vi "Sensors Page Facade.vi"(0 "Data In":T4, 2 "Display State In":T2, 3 "Container State":T3) -> (6 "Data Out":T4, 7 "Display State Out":T2, 8 "Action":T1)   [LabVIEW 2013, in "Sensors Page X.xctl"]
uses:
  Sensors Page X.xctl
  Sensors Page Data.ctl
  Sensor DAO Class.lvclass
  <vilib>/_xctls/Container State.ctl
  Sensors Page State.ctl
  <vilib>/_xctls/Action.ctl
  Sensor DAO Class.lvclass/Sensor DAO Class.ctl
  <vilib>/Utility/miscctls.llb/LVRowAndColumnTypeDef.ctl
  <vilib>/_xctls/XControlSupport.lvlib
panel:
  in  "Sensors Table":string[][](table) caption="Sensors"
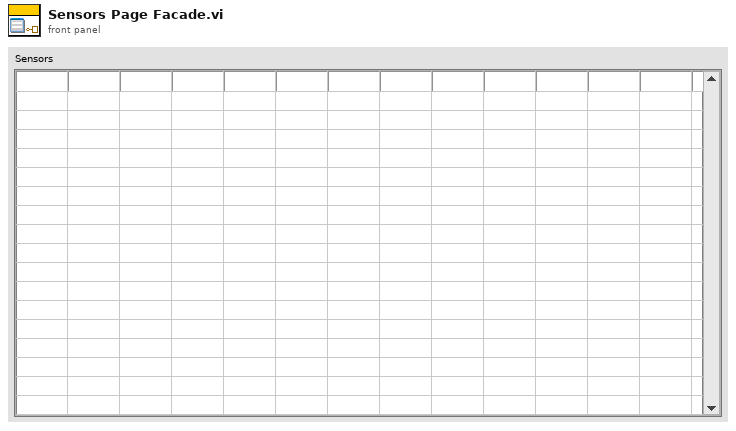
[diagram p1: front panel]
types:
  T1 = typedef "XControlSupport.lvlib/Action.ctl" = cluster{"Data Changed?":bool, "State Changed?":bool, "Action Name":string}
  T2 = typedef "Sensors Page X.xctl/Sensors Page State.ctl" = cluster{"Numeric":dbl}
  T3 = typedef "XControlSupport.lvlib/Container State.ctl" = cluster{"Indicator?":bool, "Run Mode?":bool, " Refnum":refnum<vi>}
  T4 = typedef "Sensors Page X.xctl/Sensors Page Data.ctl" = refnum<class "Sensor DAO Class.lvclass">[]
  T5 = typedef "LVRowAndColumnTypeDef.ctl" = cluster{"Row":i32, "Column":i32}
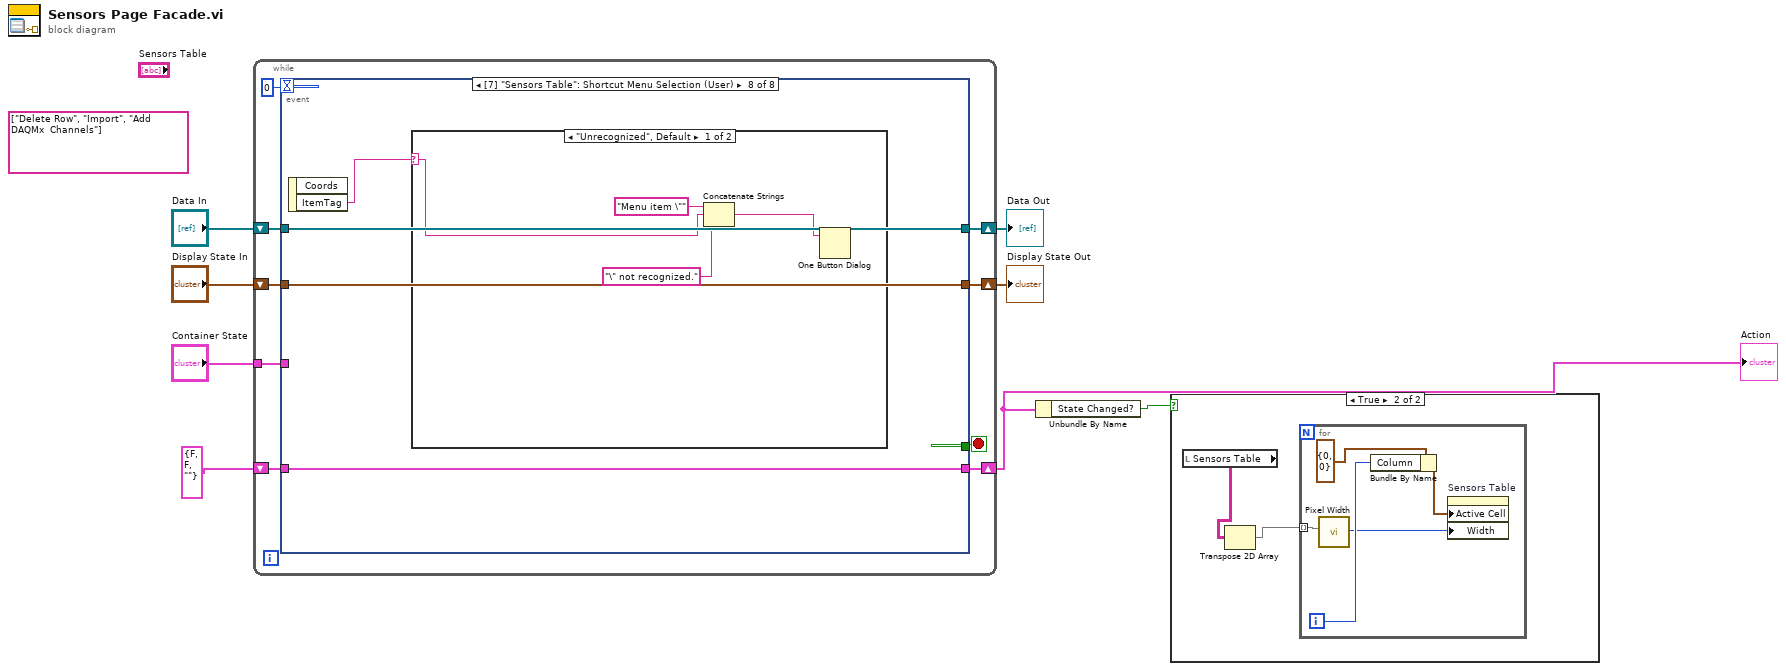
[diagram p0: block diagram]
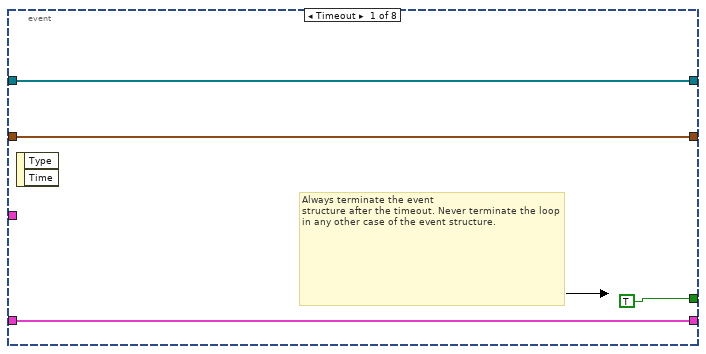
[diagram p3: hidden frame]
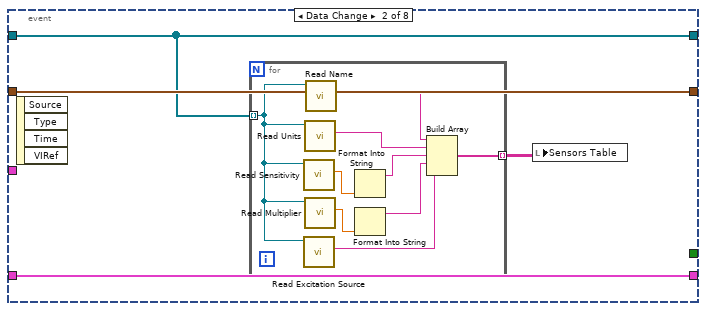
[diagram p4: hidden frame]
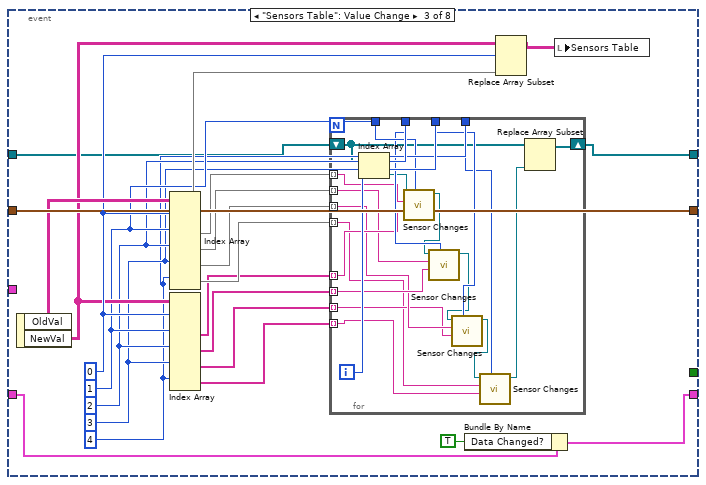
[diagram p5: hidden frame]
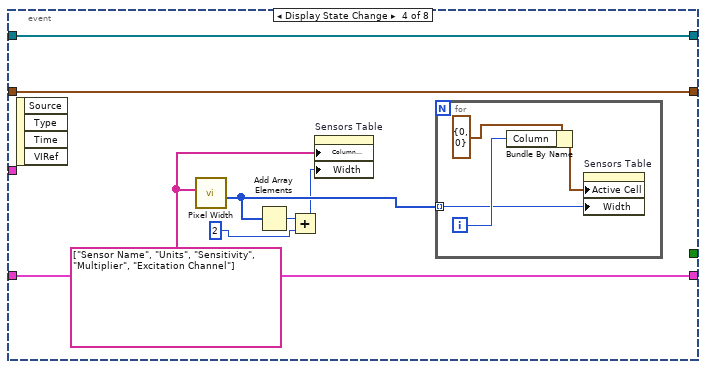
[diagram p6: hidden frame]
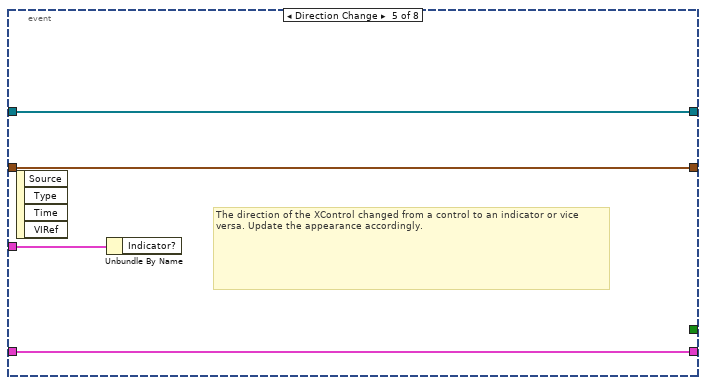
[diagram p7: hidden frame]
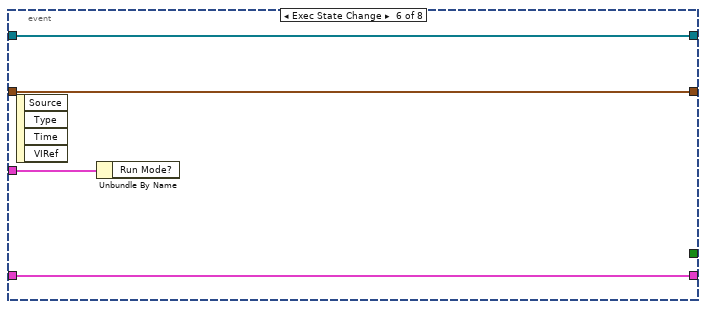
[diagram p8: hidden frame]
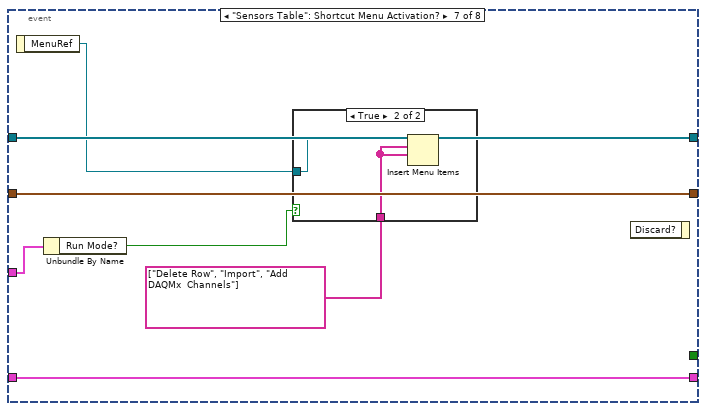
[diagram p9: hidden frame]
diagram:
  (unwired) string[] ["Delete Row", "Import", "Add DAQMx  Channels"]
  n1 = while {
    shift-right: [w16] -> w5
    shift-left: "Display State In" -> [w17]
    tunnel: "Container State" -> [w13]
    shift-right: [w11] -> w8
    shift-left: "Data In" -> [w12]
    shift-right: [w9] -> w2
    shift-left: T1 {"Data Changed?"=FALSE, "State Changed?"=FALSE, "Action Name"=""} ("Action") -> [w10]
    stop <- w15 stop-if-true
    n2 = event shown="[7] \"Sensors Table\": Shortcut Menu Selection (User)" {
      selector: _ -> [_ _ _ _ _ _ _ _]
      dyn-events: _ -> [_ _ _ _ _ _ _ _]
      timeout: 0 -> [_ _ _ _ _ _ _ _]
      tunnel: w17 -> [w19 w25 w57 w85 w92 w96 w104 w110]
      tunnel: [w19 w25 w57 w85 w92 w96 w104 w110] -> w16
      tunnel: [TRUE _ _ _ _ _ _ _] -> w15
      tunnel: w13 -> [_ _ _ _ w93 w97 w100 _]
      tunnel: w12 -> [w18 w23 w38 w84 w91 w95 w103 w109]
      tunnel: [w18 w23 w35 w84 w91 w95 w103 w109] -> w11
      tunnel: [w20 w24 w37 w83 w90 w94 w102 w108] -> w9
      tunnel: w10 -> [w20 w24 w56 w83 w90 w94 w102 w108]
      event Timeout {
        # "Always terminate the event\nstructure after the timeout. Never terminate the loop in any other case of the event structure."
        n3 = event-data() -> ()  [unwired: 1 in, 2 out]
      }
      event Data Change {
        n4 = event-data() -> ()  [unwired: 1 in, 4 out]
        n5 = for {
          tunnel: w23 -> [w34] mode=indexing
          tunnel: [w26] -> w22 mode=indexing
          n6 = call "Read Sensitivity.vi"("Sensor DAO Class in"=w34) -> ("Sensitivity"=w33:dbl)  [unwired: 8 in, 2 out]
          n7 = call "Read Excitation Source.vi"("Sensor DAO Class in"=w34) -> ("Excitation Source"=w27:string)  [unwired: 8 in, 2 out]
          n8 = call "Read Units.vi"("Sensor DAO Class in"=w34) -> ("Units"=w30:string)  [unwired: 8 in, 2 out]
          n9 = call "Read Multiplier.vi"("Sensor DAO Class in"=w34) -> ("Multiplier"=w32:dbl)  [unwired: 8 in, 2 out]
          n10 = call "Read Name.vi"("Sensor DAO Class in"=w34) -> ("Name"=w31:string)  [unwired: 8 in, 2 out]
          n11 = Format Into String(w33) -> (resulting string=w29:string)  [unwired: 3 in, 1 out]
          n12 = Format Into String(w32) -> (resulting string=w28:string)  [unwired: 3 in, 1 out]
          n13 = Build Array(w31, w30, w29, w28, w27) -> (w26:string[])
        }
        n14 = local write "Sensors Table"(w22) -> ()
      }
      event "Sensors Table": Value Change {
        w39 = 4 ("index (row)")
        w40 = 3 ("index (row)")
        w41 = 2 ("index (row)")
        w42 = 1 ("index (row)")
        w54 = 0 ("index (row)")
        n15 = event-data() -> ("OldVal"=w55:string[][], "NewVal"=w53:string[][])  [unwired: 1 in]
        n16 = Index Array(array=w55, index (row) #1=w54, index (row) #2=w42, index (row) #3=w41, index (row) #4=w40, index (row) #5=w39) -> (element #1=w52:string[], element #2=w50:string[], element #3=w49:string[], element #4=w48:string[], element #5=w47:string[])  [unwired: 5 in]
        n17 = Index Array(array=w53, index (row) #1=w54, index (row) #2=w42, index (row) #3=w41, index (row) #4=w40, index (row) #5=w39) -> (element #2=w46:string[], element #3=w45:string[], element #4=w44:string[], element #5=w43:string[])  [unwired: 5 in, 1 out]
        n18 = for {
          tunnel: w50 -> [w65] mode=indexing
          tunnel: w49 -> [w63] mode=indexing
          tunnel: w48 -> [w61] mode=indexing
          tunnel: w47 -> [w59] mode=indexing
          tunnel: w46 -> [w64] mode=indexing
          tunnel: w45 -> [w62] mode=indexing
          tunnel: w44 -> [w60] mode=indexing
          tunnel: w43 -> [w58] mode=indexing
          tunnel: w42 -> [w77]
          tunnel: w41 -> [w76]
          tunnel: w40 -> [w75]
          tunnel: w39 -> [w74]
          shift-right: [w71] -> w35
          shift-left: w38 -> [w72]
          i -> [w73]
          n19 = Index Array(array=w72, index=w73) -> (element=w70:refnum<class "Sensor DAO Class.lvclass">)
          n20 = call "Sensor Changes.vi"("Index"=w77, "New"=w64, "Old"=w65, "Sensor DAO Class In"=w70) -> ("Sensor DAO Class Out"=w69:refnum<class "Sensor DAO Class.lvclass">)  [unwired: 7 in]
          n21 = call "Sensor Changes.vi"("Index"=w76, "New"=w62, "Old"=w63, "Sensor DAO Class In"=w69) -> ("Sensor DAO Class Out"=w68:refnum<class "Sensor DAO Class.lvclass">)  [unwired: 7 in]
          n22 = call "Sensor Changes.vi"("Index"=w75, "New"=w60, "Old"=w61, "Sensor DAO Class In"=w68) -> ("Sensor DAO Class Out"=w67:refnum<class "Sensor DAO Class.lvclass">)  [unwired: 7 in]
          n23 = call "Sensor Changes.vi"("Index"=w74, "New"=w58, "Old"=w59, "Sensor DAO Class In"=w67) -> ("Sensor DAO Class Out"=w66:refnum<class "Sensor DAO Class.lvclass">)  [unwired: 7 in]
          n24 = Replace Array Subset(array=w72, new element=w66) -> (w71:T4)  [unwired: 1 in]
        }
        n25 = Bundle By Name(cluster=w56, "Data Changed?"=TRUE) -> (w37:T1)
        n26 = Replace Array Subset(array=w53, new element=w52, index (row)=w54) -> (w51:string[][])  [unwired: 1 in]
        n27 = local write "Sensors Table"(w51) -> ()
      }
      event Display State Change {
        w82 = string[] ["Sensor Name", "Units", "Sensitivity", "Multiplier", "Excitation Channel"]
        n28 = event-data() -> ()  [unwired: 1 in, 4 out]
        n29 = call "Pixel Width.vi"("Array"=w82) -> ("Widths"=w81:i32[])  [unwired: 9 in, 1 out]
        n30 = Add Array Elements(numeric array=w81) -> (sum=w80:i32)
        n31 = Add(x=w80, y=2) -> (x+y=w78:i32)
        n32 = property on="Sensors Table" class="Tbl (strict)"("Column Headers[]"=w82, "Width"=w78) -> ()  [unwired: 2 in, 2 out]
        n33 = for {
          tunnel: w81 -> [w86] mode=indexing
          i -> [w87]
          n34 = Bundle By Name(cluster=T5 {"Row"=0, "Column"=0} ("Active Cell:Active Cell"), "Column"=w87) -> (w88:T5)
          n35 = property on="Sensors Table" class="Tbl (strict)"("Active Cell"=w88, "Width"=w86) -> ()  [unwired: 2 in, 2 out]
        }
      }
      event Direction Change {
        # "The direction of the XControl changed from a control to an indicator or vice versa. Update the appearance accordingly."
        n36 = event-data() -> ()  [unwired: 1 in, 4 out]
        n37 = Unbundle By Name(w93) -> ()  [unwired: 1 out]
      }
      event Exec State Change {
        n38 = event-data() -> ()  [unwired: 1 in, 4 out]
        n39 = Unbundle By Name(w97) -> ()  [unwired: 1 out]
      }
      event "Sensors Table": Shortcut Menu Activation? {
        n40 = event-data() -> ("MenuRef"=w99:refnum<k9>)  [unwired: 1 in]
        n41 = Unbundle By Name(w100) -> ("Run Mode?"=w101:bool)
        n42 = case shown="True" w101 {
          tunnel: w99 -> [_ w106]
          tunnel: string[] ["Delete Row", "Import", "Add DAQMx  Channels"] -> [_ w105]
          frame False {
          }
          frame True {
            n43 = Insert Menu Items(7:w105, 8:w105, 9:w106) -> ()  [unwired: 3 in, 3 out]
          }
        }
        n44 = event-data() -> ()  [unwired: 2 in, 1 out]
      }
      event "Sensors Table": Shortcut Menu Selection (User) {
        n45 = event-data() -> ("ItemTag"=w107:string)  [unwired: 1 in, 1 out]
        n46 = case shown="\"Unrecognized\", Default" w107 {
          selector: w107 -> [w111 _]
          frame "Unrecognized", Default {
            n47 = Concatenate Strings("Menu item \"" ("string"), w111, "\" not recognized." ("string")) -> (w114:string)
            n48 = One Button Dialog(message=w114) -> ()  [unwired: 1 in, 1 out]
          }
          frame "True" {
          }
        }
      }
    }
  }
  "Display State Out" <- w5
  "Data Out" <- w8
  "Action" <- w2
  n49 = Unbundle By Name(w2) -> ("State Changed?"=w1:bool)
  n50 = case shown="True" w1 {
    frame False {
    }
    frame True {
      n51 = local read "Sensors Table"() -> (w116:string[][])
      n52 = Transpose 2D Array(2D array=w116) -> (transposed array=w115:string[][])
      n53 = for {
        tunnel: w115 -> [w121] mode=indexing
        i -> [w118]
        n54 = call "Pixel Width.vi"("Array"=w121) -> ("Pixel Width"=w117:i32)  [unwired: 9 in, 1 out]
        n55 = Bundle By Name(cluster=T5 {"Row"=0, "Column"=0} ("Active Cell:Active Cell"), "Column"=w118) -> (w119:T5)
        n56 = property on="Sensors Table" class="Tbl (strict)"("Active Cell"=w119, "Width"=w117) -> ()  [unwired: 2 in, 2 out]
      }
    }
  }
